vi "MSEncoder SubVI SignalRemarksAddNew_mzTable.vi"(8 "Scan time":dbl, 9 "mzTable":cluster{"t":dbl[], "mz":dbl[], "beta":dbl[]}, 10 "Label":string, 11 "MSEncoder in":refnum<class "MSEncoder.lvclass">) -> (3 "MSEncoder out":refnum<class "MSEncoder.lvclass">, 5 "Len":u32)   [LabVIEW 2018, in "MSEncoder.lvclass"]
uses:
  MSEncoder.lvclass
  PublicSubVI/Class/SigInfo/SigInfo.ctl
  MSEncoder.lvclass/MSEncoder.ctl
  PublicSubVI/Class/SigInfo/SigInfo.lvclass
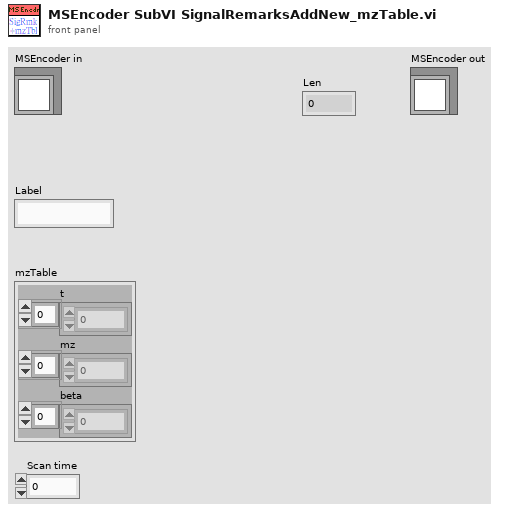
[diagram p1: front panel]
types:
  T1 = typedef "SigInfo.ctl" = enum16{"New mzList", "Set SigInfo", "Get SigInfo", "Append", "End"}
  T2 = cluster{"Label":string, "dt":dbl, "Length":u32, "RefVolt":dbl, "mzTable":cluster{"t":dbl[], "mz":dbl[], "mz 2":dbl[]}}
  T3 = cluster{"Label":string, "dt":dbl, "Length":u32, "RefVolt":dbl, "mzTable":cluster{"t":dbl[], "mz":dbl[], "beta":dbl[]}}[]
  T4 = cluster{"Label":string, "dt":dbl, "Length":u32, "RefVolt":dbl, "mzTable":cluster{"t":dbl[], "mz":dbl[], "mz 2":dbl[]}}[]
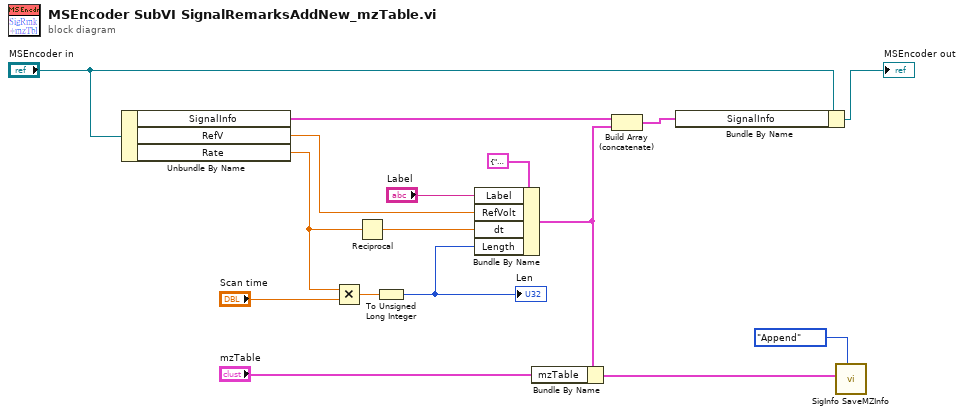
[diagram p0: block diagram]
diagram:
  n1 = Unbundle By Name("MSEncoder in") -> ("SignalInfo"=w7:T3, "RefV"=w9:dbl, "Rate"=w16:dbl)
  n2 = Multiply(x=w16, y="Scan time") -> (x*y=w15:dbl)
  n3 = Reciprocal(x=w16) -> (1/x=w12:dbl)
  n4 = To Unsigned Long Integer(number=w15) -> (unsigned 32bit integer=w11:u32)
  "Len" <- w11
  n5 = Bundle By Name(cluster=T2 {"Label"="", "dt"=0.0, "Length"=0, "RefVolt"=0.0, "mzTable"={"t"=[], "mz"=[], "mz 2"=[]}} ("SigInfo"), "Label"="Label", "RefVolt"=w9, "dt"=w12, "Length"=w11) -> (w4:T2)
  n6 = Bundle By Name(cluster=w4, "mzTable"="mzTable") -> (w3:T2)
  n7 = Build Array (concatenate)(w7, w4) -> (w6:T4)
  n8 = Bundle By Name(cluster="MSEncoder in", "SignalInfo"=w6) -> (→"MSEncoder out":refnum<class "MSEncoder.lvclass">)
  n9 = call "SigInfo SaveMZInfo.vi"("Function"=SigInfo."Append", "SigInfo"=w3) -> ()  [unwired: 7 in, 3 out]
